vi "closeCameraServer.vi"(8 "error in (no error)":errorcluster, 11 "CameraNetworkController in":refnum<class "CameraNetworkController.lvclass">) -> (0 "error out":errorcluster)   [LabVIEW 2009, in "Hardware.lvlib" / "HWControllers.lvlib" / "CameraNetworkController.lvclass"]
uses:
  CameraNetworkController.lvclass
  NetworkClient/NetworkServer.lvclass
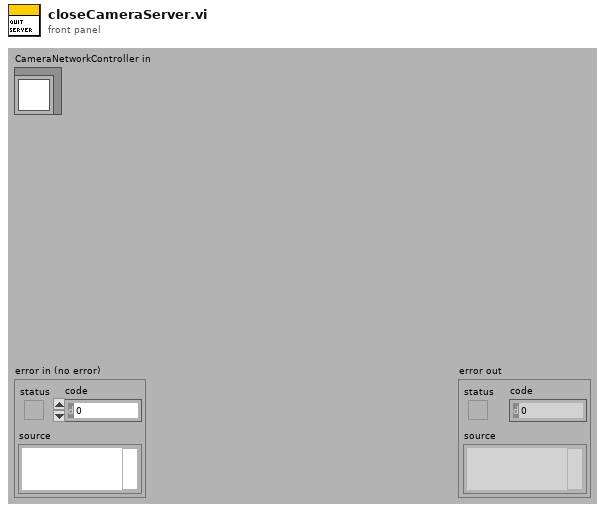
[diagram p1: front panel]
types:
  T1 = cluster{"Message":enum16{"Idle", "initialise", "configureAcquisition", "setTemperature", "getTemperature", "start", "stop", "sendImage", "close", "error", "ExitApp"}, "Data":variant}
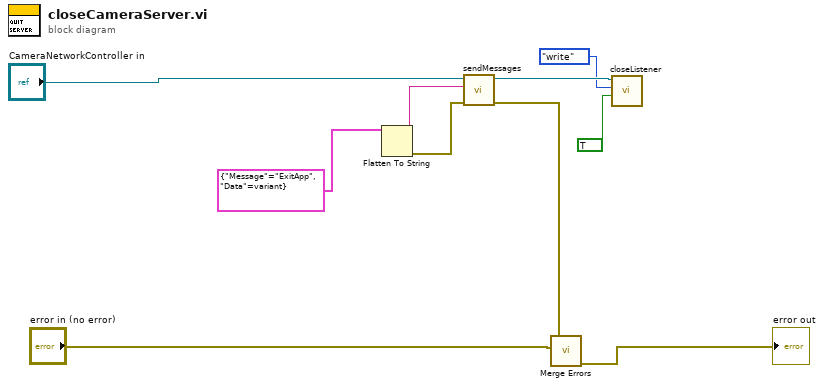
[diagram p0: block diagram]
diagram:
  n1 = Flatten To String(anything=T1 {"Message"=enum."ExitApp", "Data"=variant}) -> (data string=w8:string, error out=w7:errorcluster)  [unwired: 3 in, 1 out]
  n2 = call "sendMessages.vi"("error in (no error)"=w7, "messageString"=w8, "NetworkClient in"="CameraNetworkController in") -> ("error out"=w3:errorcluster, "NetworkClient out"=w6:refnum<class "CameraNetworkController.lvclass">)  [unwired: 7 in]
  n3 = call <vilib>:"Merge Errors.vi"("error in 2 (no error)"="error in (no error)", "error in 1 (no error)"=w3) -> ("error out"=→"error out":errorcluster)  [unwired: 5 in]
  n4 = call "closeListener.vi"("close"=TRUE, "actions"=enum16{"read", "write"}."write", "NetworkServer in"=w6) -> ()  [unwired: 6 in, 3 out]
